vi "Analysis.LevelTransition.vi"(8 "error in":errorcluster, 10 "Result.Prefix":string="Result.", 11 "tdms file":refnum<k34>) -> (0 "error out":errorcluster, 3 "tdms file out":refnum<k34>)   [LabVIEW 2015, in "TestStand Analysis Steps.lvlib"]
uses:
  TestStand Analysis Steps.lvlib
  SubVIs/Analysis.SingleChannelLevelTransitionLogic.vi
  Shared/Constants.vi
  Shared/Shared.lvlib
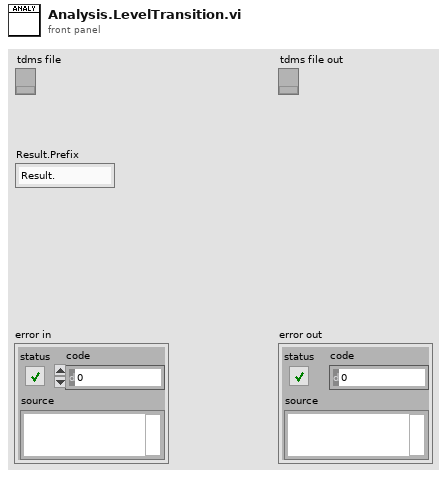
[diagram p1: front panel]
types:
  T1 = typedef "Shared.lvlib/Public.LVAnalysis.ctl" = cluster{"ODH":T2, "OPH.Duty":T2, "OPH.Freq":T2}
  T2 = typedef "Shared.lvlib/Public.ChLVAnalysis.ctl" = cluster{"Level":dbl, "Band":dbl, "TimeTolerance":dbl}
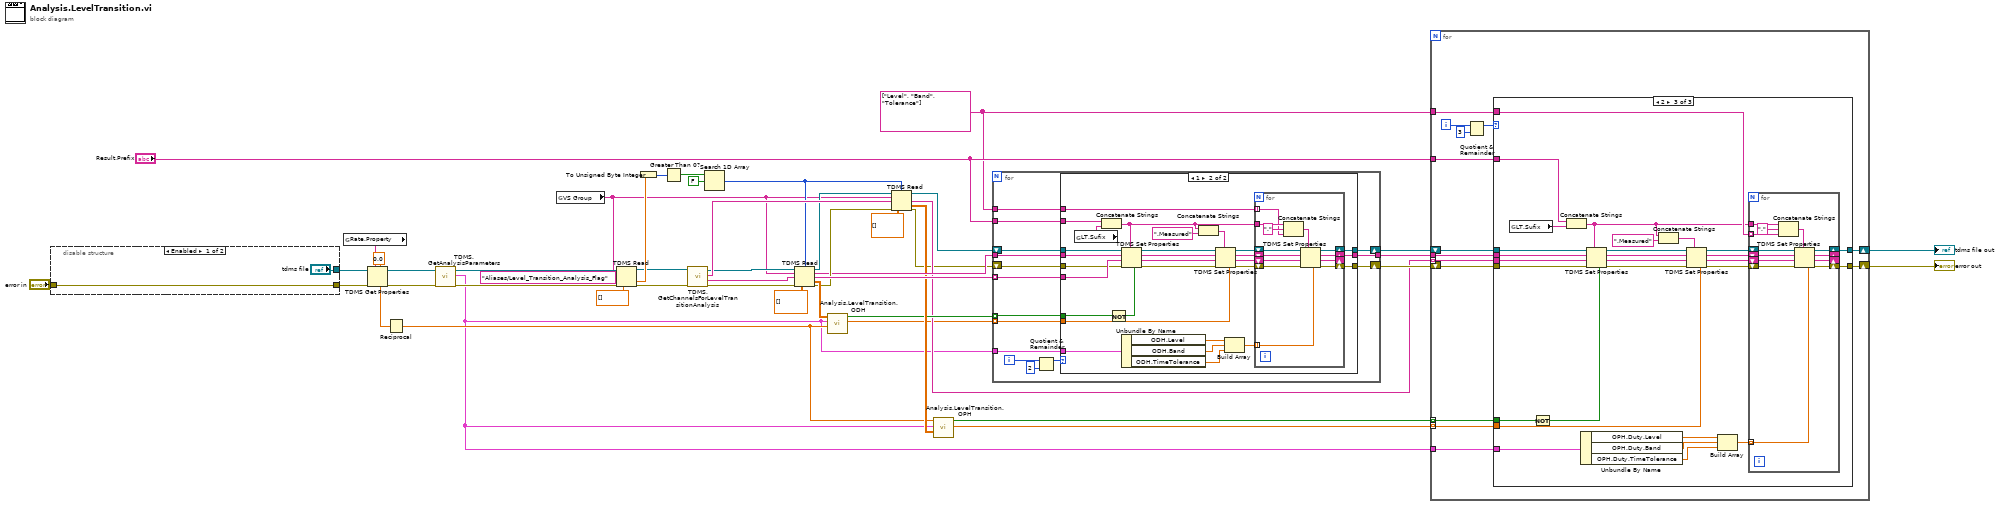
[diagram p0: block diagram]
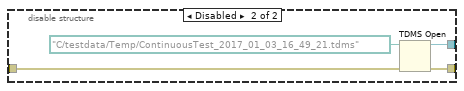
[diagram p3: hidden frame]
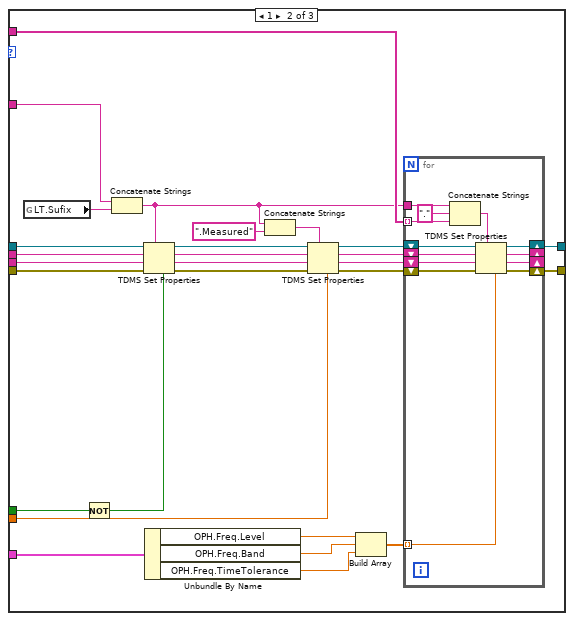
[diagram p5: hidden frame]
diagram:
  w1 = string[] ["Level", "Band", "Tolerance"]
  n1 = disable-structure shown="Enabled" {
    disable-tunnel: ["tdms file" w53] -> w13
    disable-tunnel: "error in" -> [w49 w52]
    disable-tunnel: [w49 w51] -> w9
    frame Enabled {
    }
    frame Disabled {
      n2 = TDMS Open(8:w52, 11:path "C:/testdata/Temp/ContinuousTest_2017_01_03_16_49_21.tdms" ("file path")) -> (0:w51:errorcluster, 3:w53:refnum<k34>)  [unwired: 5 in]
    }
  }
  n3 = global read "Constants.vi" "Rate.Property"() -> (w8:string)
  n4 = TDMS Get Properties(5:0.0, 7:w8, 8:w9, 11:w13) -> (0:w20:errorcluster, 3:w21:refnum<k34>, 4:w46:dbl)  [unwired: 2 in, 3 out]
  n5 = Reciprocal(x=w46) -> (1/x=w36:dbl)
  n6 = call "TDMS.GetAnalysisParameters.vi"("error in (no error)"=w20, "TDMS Ref"=w21) -> ("error out"=w23:errorcluster, "LVTransitionParameters"=w7:T1, "TDMS Ref"=w22:refnum<k34>)  [unwired: 6 in, 1 out]
  n7 = global read "Constants.vi" "VS Group"() -> (w12:string)
  n8 = TDMS Read(0:w22, 5:w12, 7:"Aliases/Level_Transition_Analysis_Flag" ("channel name(s) in"), 11:w23, 12:dbl[] []) -> (4:w24:refnum<k34>, 10:w32:dbl[], 15:w25:errorcluster)  [unwired: 3 in, 3 out]
  n9 = To Unsigned Byte Integer(number=w32) -> (unsigned 8bit integer=w31:u8[])
  n10 = Greater Than 0?(x=w31) -> (x > 0?=w30:bool[])
  n11 = call "TDMS.GetChannelsForLevelTransitionAnalysis.vi"("error in (no error)"=w25, "TDMS Ref"=w24) -> ("error out"=w27:errorcluster, "ODH Channels"=w14:string[], "OPH Channels"=w41:string[], "TDMS Ref out"=w26:refnum<k34>)  [unwired: 6 in]
  n12 = Search 1D Array(1D array=w30, element=FALSE) -> (index of element=w28:i32)  [unwired: 1 in]
  n13 = TDMS Read(0:w26, 2:w28, 5:w12, 7:w14, 11:w27, 12:dbl[][] []) -> (4:w37:refnum<k34>, 6:w42:string, 8:w44:string[], 10:w45:dbl[][], 15:w43:errorcluster)  [unwired: 2 in, 1 out]
  n14 = call "Analysis.LevelTransition.ODH.vi"("Numeric"=w36, "LVTransitionParameters"=w7, "Array in"=w45) -> ("Results"=w3:dbl[], "Array out"=w38:bool[])  [unwired: 7 in]
  n15 = TDMS Read(0:w37, 2:w28, 5:w12, 7:w41, 11:w43, 12:dbl[][] []) -> (4:w4:refnum<k34>, 8:w15:string[], 10:w39:dbl[][], 15:w5:errorcluster)  [unwired: 2 in, 2 out]
  n16 = call "Analysis.LevelTransition.OPH.vi"("Array in"=w39, "LVTransitionParameters"=w7, "Numeric"=w36) -> ("Results"=w2:dbl[], "Array out"=w16:bool[])  [unwired: 7 in]
  n17 = for {
    tunnel: w38 -> [w67] mode=indexing
    tunnel: w44 -> [w66] mode=indexing
    shift-right: [w63] -> w18
    shift-left: w5 -> [w65]
    shift-right: [w62] -> w19
    shift-left: w4 -> [w69]
    tunnel: w42 -> [w68]
    tunnel: [w61] -> w17
    tunnel: "Result.Prefix" -> [w64]
    tunnel: w7 -> [w60]
    tunnel: w1 -> [w59]
    tunnel: w3 -> [w58] mode=indexing
    i -> [w56]
    n18 = Quotient & Remainder(x=w56, y=2) -> (x-y*floor(x/y)=w55:i32)  [unwired: 1 out]
    n19 = case shown="1" w55 {
      tunnel: w69 -> [w72 w101]
      tunnel: w68 -> [w71 w100]
      tunnel: w67 -> [_ w98]
      tunnel: w66 -> [_ w97]
      tunnel: w65 -> [w70 w96]
      tunnel: w64 -> [_ w95]
      tunnel: [w70 w93] -> w63
      tunnel: [w72 w92] -> w62
      tunnel: [w71 w91] -> w61
      tunnel: w60 -> [_ w90]
      tunnel: w59 -> [_ w89]
      tunnel: w58 -> [_ w84]
      frame 0, Default {
      }
      frame 1 {
        n20 = global read "Constants.vi" "LT.Sufix"() -> (w94:string)
        n21 = Concatenate Strings(w95, w94) -> (w83:string)
        n22 = Not(x=w98) -> (.not. x?=w99:bool)
        n23 = Unbundle By Name(w90) -> ("ODH.Level"=w82:dbl, "ODH.Band"=w81:dbl, "ODH.TimeTolerance"=w80:dbl)
        n24 = TDMS Set Properties(5:w99, 7:w83, 8:w96, 9:w97, 10:w100, 11:w101) -> (0:w88:errorcluster, 1:w87:string, 2:w86:string, 3:w85:refnum<k34>)
        n25 = Concatenate Strings(w83, ".Measured" ("string")) -> (w73:string)
        n26 = TDMS Set Properties(5:w84, 7:w73, 8:w88, 9:w87, 10:w86, 11:w85) -> (0:w78:errorcluster, 1:w77:string, 2:w76:string, 3:w75:refnum<k34>)
        n27 = Build Array(w82, w81, w80) -> (w79:dbl[])
        n28 = for {
          tunnel: w83 -> [w108]
          shift-right: [w111] -> w93
          shift-left: w78 -> [w114]
          shift-right: [w110] -> w92
          shift-left: w75 -> [w113]
          shift-right: [w109] -> w91
          shift-left: w76 -> [w112]
          tunnel: w79 -> [w105] mode=indexing
          tunnel: w89 -> [w104] mode=indexing
          shift-right: [w102] -> _
          shift-left: w77 -> [w103]
          n29 = Concatenate Strings(w108, "." ("string"), w104) -> (w106:string)
          n30 = TDMS Set Properties(5:w105, 7:w106, 8:w114, 9:w103, 10:w112, 11:w113) -> (0:w111:errorcluster, 1:w102:string, 2:w109:string, 3:w110:refnum<k34>)
        }
      }
    }
  }
  n31 = for {
    tunnel: w16 -> [w116] mode=indexing
    tunnel: w15 -> [w117] mode=indexing
    shift-right: [w126] -> w10
    shift-left: w18 -> [w120]
    shift-right: [w125] -> w11
    shift-left: w19 -> [w119]
    tunnel: w17 -> [w118]
    tunnel: "Result.Prefix" -> [w115]
    tunnel: w7 -> [w128]
    tunnel: w1 -> [w127]
    tunnel: w2 -> [w122] mode=indexing
    i -> [w124]
    n32 = Quotient & Remainder(x=w124, y=3) -> (x-y*floor(x/y)=w121:i32)  [unwired: 1 out]
    n33 = case shown="2" w121 {
      tunnel: w128 -> [_ w158 w196]
      tunnel: w127 -> [_ w153 w194]
      tunnel: [w129 w152 w193] -> w126
      tunnel: [w130 w151 w192] -> w125
      tunnel: w120 -> [w129 w140 w181]
      tunnel: w119 -> [w130 w137 w178]
      tunnel: w118 -> [_ w138 w179]
      tunnel: w117 -> [_ w139 w180]
      tunnel: w115 -> [_ w132 w177]
      tunnel: w122 -> [_ w146 w187]
      tunnel: w116 -> [_ w141 w182]
      frame Default {
      }
      frame 1 {
        n34 = global read "Constants.vi" "LT.Sufix"() -> (w142:string)
        n35 = Not(x=w141) -> (.not. x?=w143:bool)
        n36 = Concatenate Strings(w132, w142) -> (w131:string)
        n37 = TDMS Set Properties(5:w143, 7:w131, 8:w140, 9:w139, 10:w138, 11:w137) -> (0:w133:errorcluster, 1:w134:string, 2:w135:string, 3:w136:refnum<k34>)
        n38 = Unbundle By Name(w158) -> ("OPH.Freq.Level"=w157:dbl, "OPH.Freq.Band"=w156:dbl, "OPH.Freq.TimeTolerance"=w155:dbl)
        n39 = Concatenate Strings(w131, ".Measured" ("string")) -> (w144:string)
        n40 = TDMS Set Properties(5:w146, 7:w144, 8:w133, 9:w134, 10:w135, 11:w136) -> (0:w150:errorcluster, 1:w148:string, 2:w147:string, 3:w149:refnum<k34>)
        n41 = Build Array(w157, w156, w155) -> (w154:dbl[])
        n42 = for {
          tunnel: w131 -> [w165]
          shift-right: [w168] -> w152
          shift-left: w150 -> [w171]
          shift-right: [w167] -> w151
          shift-left: w149 -> [w170]
          shift-right: [w166] -> _
          shift-left: w147 -> [w169]
          tunnel: w154 -> [w162] mode=indexing
          tunnel: w153 -> [w161] mode=indexing
          shift-right: [w159] -> _
          shift-left: w148 -> [w160]
          n43 = Concatenate Strings(w165, "." ("string"), w161) -> (w163:string)
          n44 = TDMS Set Properties(5:w162, 7:w163, 8:w171, 9:w160, 10:w169, 11:w170) -> (0:w168:errorcluster, 1:w159:string, 2:w166:string, 3:w167:refnum<k34>)
        }
      }
      frame 2 {
        n45 = global read "Constants.vi" "LT.Sufix"() -> (w183:string)
        n46 = Not(x=w182) -> (.not. x?=w184:bool)
        n47 = Concatenate Strings(w177, w183) -> (w176:string)
        n48 = Unbundle By Name(w196) -> ("OPH.Duty.Level"=w197:dbl, "OPH.Duty.Band"=w198:dbl, "OPH.Duty.TimeTolerance"=w199:dbl)
        n49 = TDMS Set Properties(5:w184, 7:w176, 8:w181, 9:w180, 10:w179, 11:w178) -> (0:w172:errorcluster, 1:w173:string, 2:w174:string, 3:w175:refnum<k34>)
        n50 = Concatenate Strings(w176, ".Measured" ("string")) -> (w185:string)
        n51 = TDMS Set Properties(5:w187, 7:w185, 8:w172, 9:w173, 10:w174, 11:w175) -> (0:w191:errorcluster, 1:w189:string, 2:w188:string, 3:w190:refnum<k34>)
        n52 = Build Array(w197, w198, w199) -> (w195:dbl[])
        n53 = for {
          tunnel: w176 -> [w206]
          shift-right: [w209] -> w193
          shift-left: w191 -> [w212]
          shift-right: [w208] -> w192
          shift-left: w190 -> [w211]
          shift-right: [w207] -> _
          shift-left: w188 -> [w210]
          tunnel: w195 -> [w203] mode=indexing
          tunnel: w194 -> [w202] mode=indexing
          shift-right: [w200] -> _
          shift-left: w189 -> [w201]
          n54 = Concatenate Strings(w206, "." ("string"), w202) -> (w204:string)
          n55 = TDMS Set Properties(5:w203, 7:w204, 8:w212, 9:w201, 10:w210, 11:w211) -> (0:w209:errorcluster, 1:w200:string, 2:w207:string, 3:w208:refnum<k34>)
        }
      }
    }
  }
  "error out" <- w10
  "tdms file out" <- w11
